vi "Read Coral Operation.vi"(8 "Command Info":T5) -> (0 "Command Info":T5, 1 "SubSystem Data":T1, 2 "Command Timing":cluster{"Start Time (ms)":u32, "Iterations":i32})   [LabVIEW 2023]
doc: "This returns the most recently scheduled command. This doesn't indicate whether the command finished and is running the default command."
uses:
  <vilib>/Rock Robotics/WPI/Framework/Command Status Info.ctl
  <vilib>/Rock Robotics/WPI/Framework/Completion Status.ctl
  <vilib>/Rock Robotics/WPI/Framework/Completion Notifier.ctl
  Implementation/Coral Setpoints.ctl
  Implementation/Coral Operations.ctl
  Support Code/Teleop Util/Coral States.ctl
  Support Code/Teleop Util/Scoring Levels.ctl
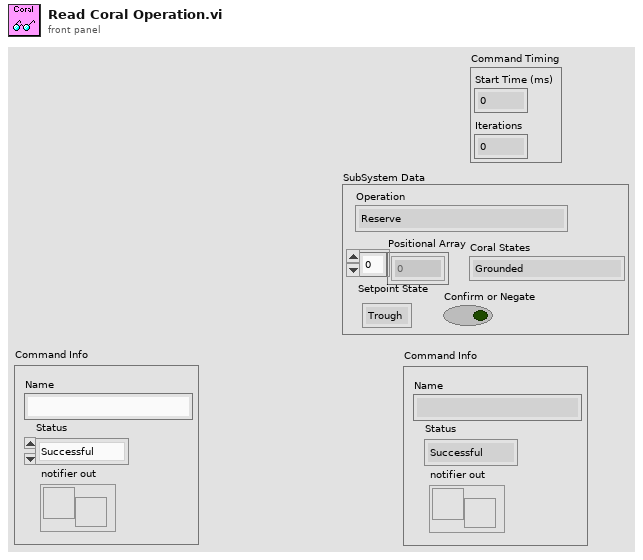
[diagram p1: front panel]
types:
  T1 = typedef "Coral Setpoints.ctl" = cluster{"Operation":T2, "Coral States":T3, "Confirm or Negate":bool, "Positional Array":dbl[], "Setpoint State":T4}
  T2 = typedef "Coral Operations.ctl" = enum16{"Reserve", "Read Current", "Immediate", "Calibrate"}
  T3 = typedef "Coral States.ctl" = enum16{"Grounded", "Coral Intake", "Scoring Sequence", "Hold Position", "Score", "Manual Override", "Climb Safety Mode"}
  T4 = typedef "Scoring Levels.ctl" = enum16{"Trough", "L2", "L3", "L4", "Default"}
  T5 = typedef "Command Status Info.ctl" = cluster{"Name":string, "Status":T6, "notifier out":T7}
  T6 = typedef "Completion Status.ctl" = enum16{"Successful", "Aborted", "Incomplete"}
  T7 = typedef "Completion Notifier.ctl" = refnum<notifier>
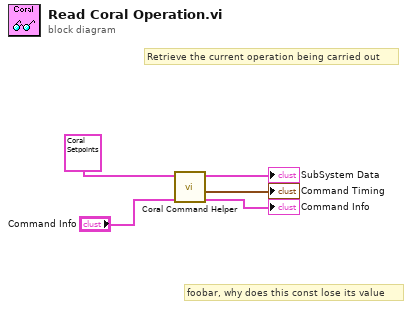
[diagram p0: block diagram]
diagram:
  # "foobar, why does this const lose its value"
  # "Retrieve the current operation being carried out"
  n1 = call "Coral Command Helper.vi"("Command Info In"="Command Info", "SubSystem Data"=T1 {"Operation"=enum."Read Current", "Coral States"=enum."Grounded", "Confirm or Negate"=FALSE, "Positional Array"=[], "Setpoint State"=enum."L4"}) -> ("Command Info Out"=→"Command Info":T5, "Command Timing"=→"Command Timing":cluster{"Start Time (ms)":u32, "Iterations":i32}, "SubSystem Data"=→"SubSystem Data":T1)  [unwired: 7 in]
